vi "SampleCode.vi"() -> ()   [LabVIEW 2016]
uses:
  uPythonX/uPythonX.xctl
panel:
  out "Console":string
  in  "stop":bool
  in  "uPythonX":T1(xcontrol)
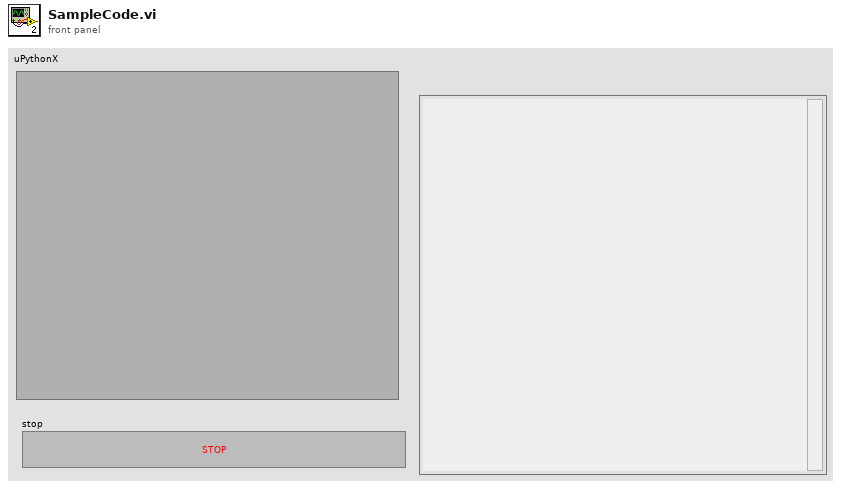
[diagram p1: front panel]
types:
  T1 = cluster{"VISA Refnum in":refnum<visa-resource-name>, "Python Code":string}
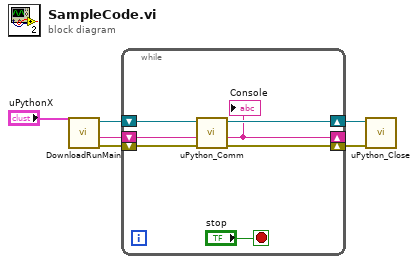
[diagram p0: block diagram]
diagram:
  n1 = call "DownloadRunMain.vi"("Data In"="uPythonX") -> ("error out"=w5:errorcluster, "Reply"=w4:string, "VISA Refnum out"=w3:refnum<visa-resource-name>)  [unwired: 8 in]
  n2 = while {
    shift-right: [w10] -> w2
    shift-left: w5 -> [w13]
    shift-right: [w9] -> w1
    shift-left: w3 -> [w11]
    shift-right: [w7] -> _
    shift-left: w4 -> [w12]
    stop <- "stop" stop-if-true
    n3 = call "uPython_Comm.vi"("error in (no error)"=w13, "Console In"=w12, "VISA Refnum in"=w11) -> ("error out"=w10:errorcluster, "Console Out"=w7:string, "VISA out"=w9:refnum<visa-resource-name>)  [unwired: 4 in, 2 out]
    "Console" <- w7
  }
  n4 = call "uPython_Close.vi"("error in"=w2, "VISA  in"=w1) -> ()  [unwired: 8 in, 2 out]
